vi "select_previous_roi.vi"(6 "title in":string="2010_10_15__14_02_52", 8 "error in":errorcluster, 11 "times in":string[](array[string])) -> (0 "error out":errorcluster, 3 "selector out":i32)   [LabVIEW 2010, in "TrajectoryMH100122AODRAPS.lvclass"]
uses:
  TrajectoryMH100122AODRAPS.lvclass
panel:
  in  "array of boolean":bool[](array[boolean])
  # "Select the ROI time stamp to recover the ROIs from the file."
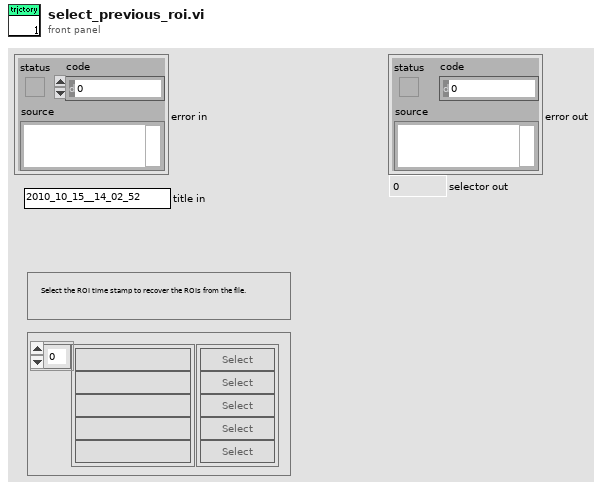
[diagram p1: front panel]
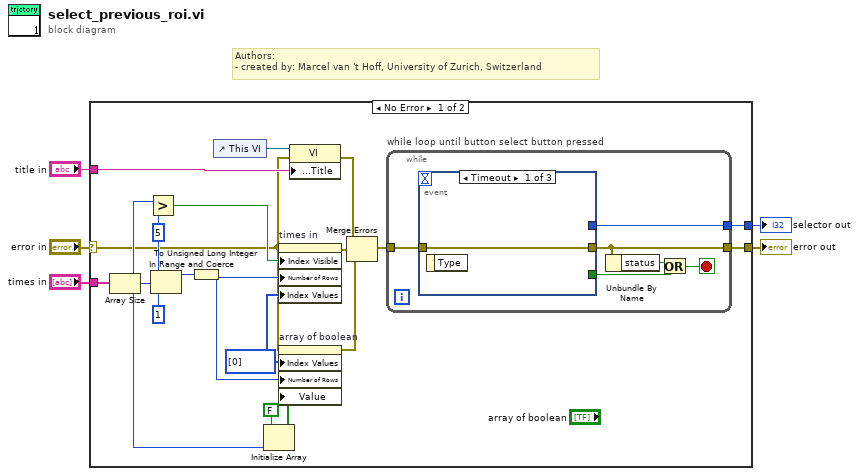
[diagram p0: block diagram]
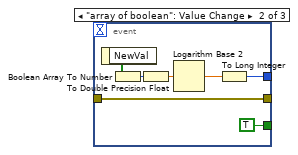
[diagram p2: hidden frame]
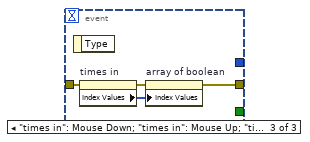
[diagram p3: hidden frame]
diagram:
  # "Authors: \n- created by: Marcel van 't Hoff, University of Zurich, Switzerland"
  n1 = case shown="No Error" "error in" {
    selector: "error in" -> [w7 w43]
    tunnel: "times in" -> [w23 _]
    tunnel: [w11 w43] -> w4
    tunnel: [w10 _] -> w3
    tunnel: "title in" -> [w8 _]
    frame No Error {
      w15 = u32[] [0] ("Index Values")
      w18 = 5 ("upper limit")
      n2 = Array Size(array=w23) -> (size(s)=w16:i32)
      n3 = Greater?(x=w16, y=w18) -> (0:w17:bool)
      n4 = In Range and Coerce(upper limit=w18, x=w16, lower limit=1) -> (coerced(x)=w19:i32)  [unwired: 1 out]
      n5 = To Unsigned Long Integer(number=w19) -> (unsigned 32bit integer=w21:u32)
      n6 = control-ref of="This VI"() -> (w9:refnum<vi>)
      n7 = Initialize Array(FALSE, w16) -> (w20:bool[])
      n8 = property on="times in" class="Arr (strict)"(error in=w7, "Index Visible"=w17, "Number of Rows"=w21, "Index Values"=w15) -> (error out=w14:errorcluster)  [unwired: 1 in, 1 out]
      n9 = property on="array of boolean" class="Arr (strict)"(error in=w7, "Index Values"=w15, "Number of Rows"=w21, "Value"=w20) -> (error out=w12:errorcluster)  [unwired: 1 in, 1 out]
      n10 = property class="VI"(reference=w9, error in=w7, "Front Panel.Title"=w8) -> (error out=w6:errorcluster)  [unwired: 1 out]
      n11 = Merge Errors(w6, w14, w12) -> (w13:errorcluster)
      n12 = while "while loop until button select button pressed" {
        tunnel: [w25] -> w10
        tunnel: w13 -> [w30]
        tunnel: [w29] -> w11
        stop <- w27 stop-if-true
        n13 = event shown="[0] Timeout" {
          selector: _ -> [_ _ _]
          dyn-events: _ -> [_ _ _]
          timeout: _ -> [_ _ _]
          tunnel: [w31 w38 w40] -> w29
          tunnel: w30 -> [w31 w38 w39]
          tunnel: [_ TRUE _] -> w26
          tunnel: [_ w32 _] -> w25
          event Timeout {
            n14 = event-data() -> ()  [unwired: 1 in, 1 out]
          }
          event "array of boolean": Value Change {
            n15 = event-data() -> ("NewVal"=w34:bool[])  [unwired: 1 in]
            n16 = Boolean Array To Number(Boolean array=w34) -> (number=w37:u32)
            n17 = To Double Precision Float(number=w37) -> (double precision float=w36:dbl)
            n18 = Logarithm Base 2(1:w36) -> (0:w33:dbl)
            n19 = To Long Integer(number=w33) -> (32bit integer=w32:i32)
          }
          event "times in": Mouse Down; "times in": Mouse Up; "times in": Key Down; "times in": Key Up {
            n20 = event-data() -> ()  [unwired: 1 in, 1 out]
            n21 = property on="times in" class="Arr (strict)"(error in=w39) -> (error out=w41:errorcluster, "Index Values"=w42:u32[])  [unwired: 1 in, 1 out]
            n22 = property on="array of boolean" class="Arr (strict)"(error in=w41, "Index Values"=w42) -> (error out=w40:errorcluster)  [unwired: 1 in, 1 out]
          }
        }
        n23 = Unbundle By Name(w29) -> ("status"=w28:bool)
        n24 = Or(x=w28, y=w26) -> (x .or. y?=w27:bool)
      }
    }
    frame Error {
    }
  }
  "error out" <- w4
  "selector out" <- w3
